vi "Terminal_Global_User_name.vi"() -> ()   [LabVIEW 2014]
panel:
  out "用户名":string
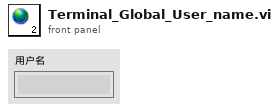
[diagram p1: front panel]
diagram:
